vi "室内外单幅图像-视频预览.vi"() -> ()   [LabVIEW 2018]
doc: "This example shows how to open, read, and display an AVI file in NI Vision. The VI reads the frames per second property and plays the images back at the rate specified by the AVI file."
uses:
  <vilib>/Utility/error.llb/DialogType.ctl
panel:
  out "数值输入控件":i32
  in  "重新读取":bool
  out "视频的帧数：":u32
  out "Path":path
  out "添加的路径":path
  out "视频预览":T1(plugin-control)
  in  "Stop 2":bool
  out "Progress Bar 2":i32(slide) max=25 scale=-1.0..25.0
  in  "下一步":bool
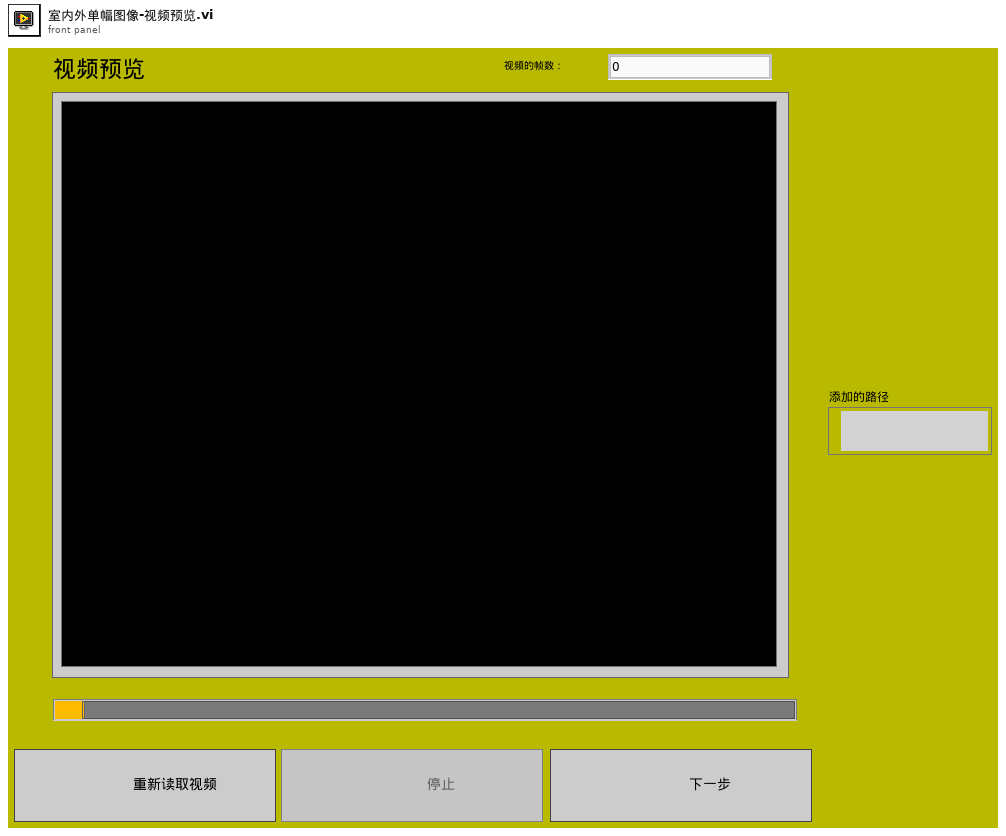
[diagram p1: front panel]
types:
  T1 = typedef "IMAQ Image.ctl" = refnum<image>
  T2 = enum8{"Enabled", "Disabled", "Disabled and Grayed Out"}
  T3 = enum32{"Invalid", "Standard", "Closed", "Hidden", "Minimized", "Maximized"}
  T4 = typedef "DialogType.ctl" = u16
  T5 = typedef "IMAQ AVI2 Refnum.ctl" = refnum<k20>
  T6 = typedef "Image Type" = u32
  T7 = cluster{"Width":u32, "Height":u32, "Frames Per Second":u32, "Codec":string, "Has Data":bool}
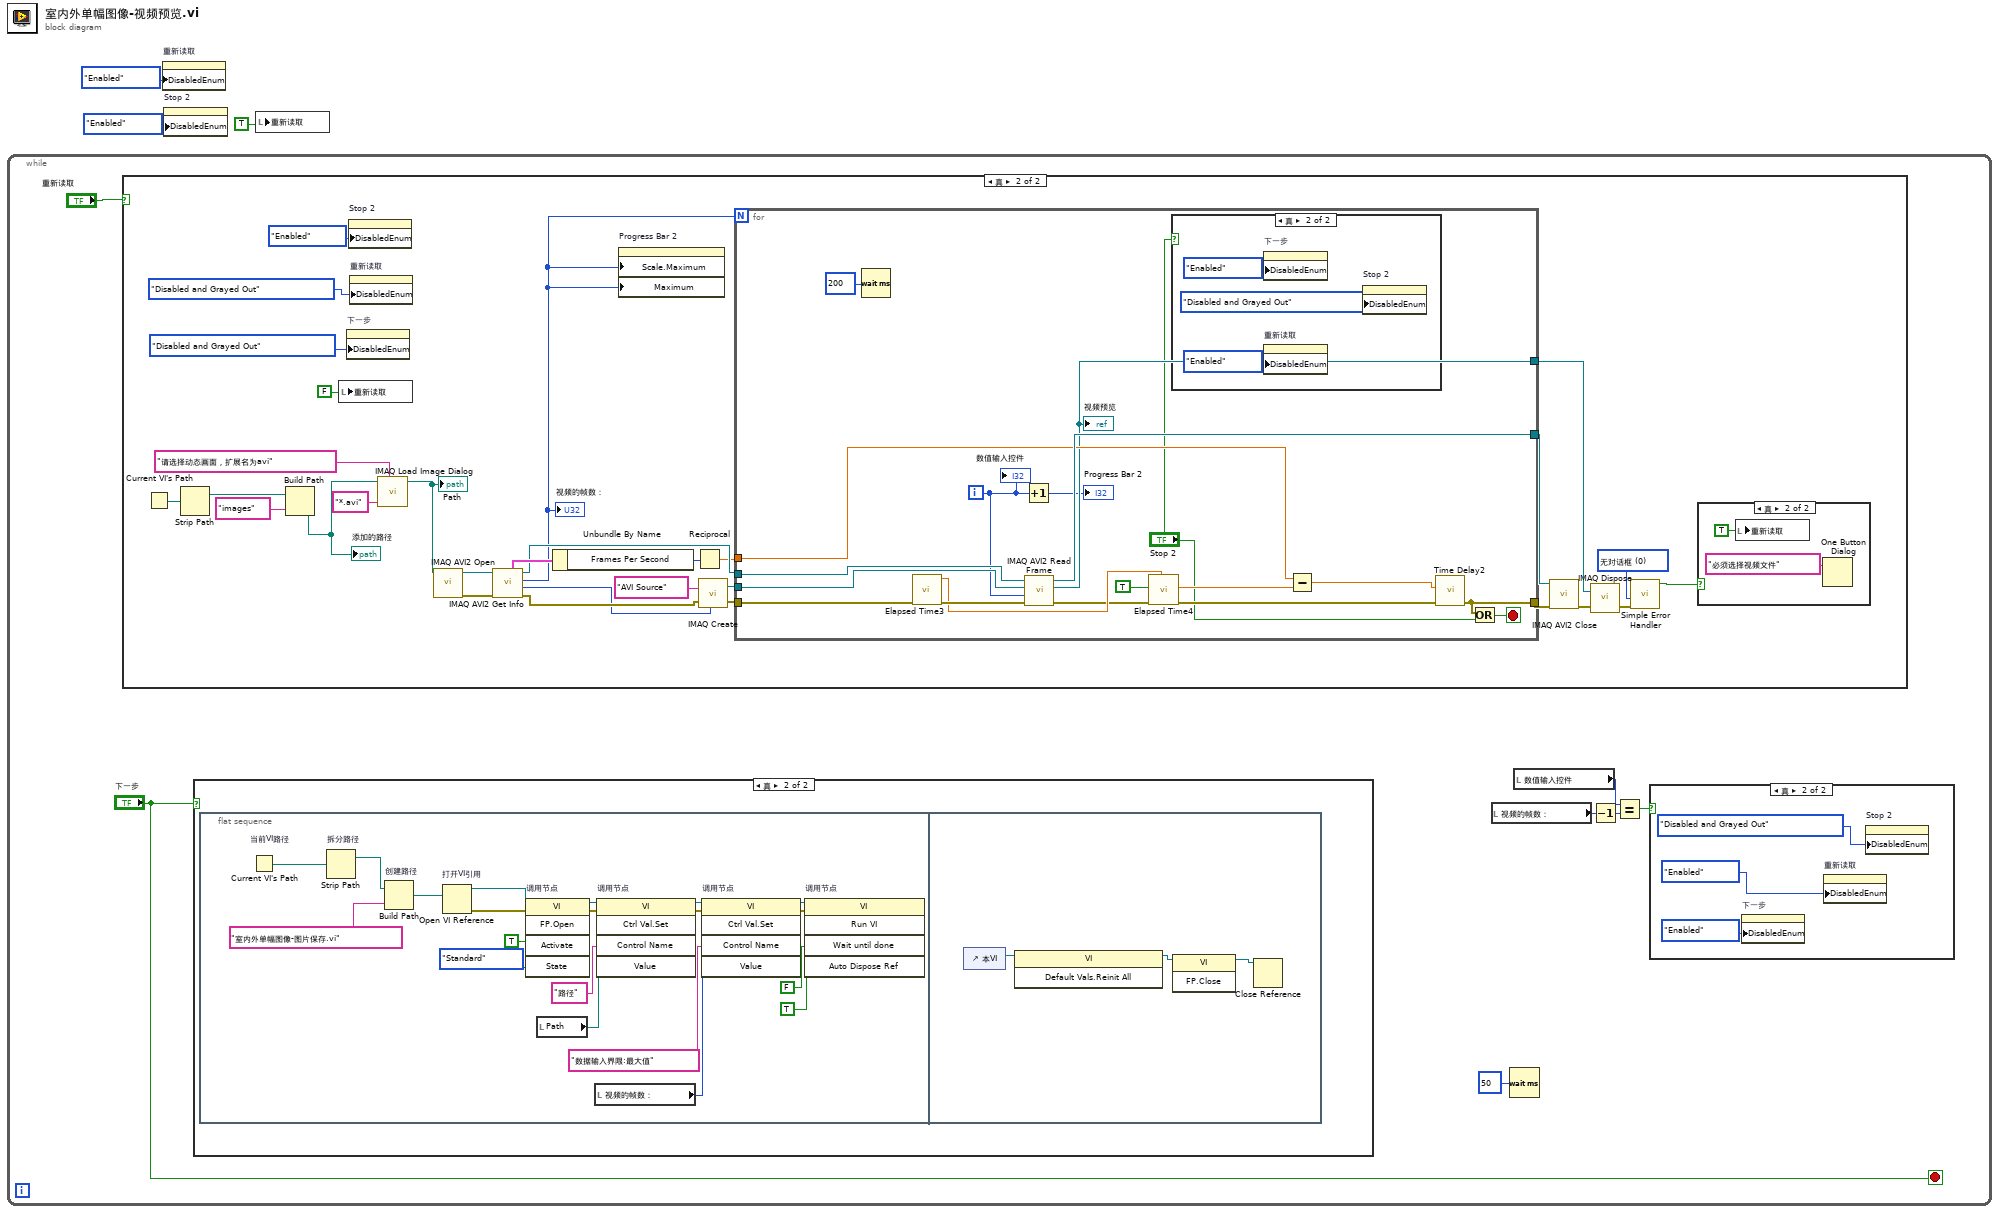
[diagram p0: block diagram]
diagram:
  n1 = while {
    stop <- "下一步" stop-if-true
    n2 = case shown="真" "重新读取" {
      frame False {
      }
      frame True {
        w19 = T4 0 items=["无对话框", "确定信息", "继续或停止信息", "确定信息＋警告", "继续/停止+警告"] ("type of dialog (OK msg:1)")
        n3 = Current VI's Path() -> (path=w23:path)
        n4 = Strip Path(path=w23) -> (stripped path=w22:path)  [unwired: 1 out]
        n5 = Build Path(base path=w22, name or relative path="images") -> (appended path=w26:path)
        "添加的路径" <- w26
        n6 = local write "重新读取"(FALSE ("布尔")) -> ()
        n7 = property on="下一步" class="Bool (严格)"("DisabledEnum"=T2."Disabled and Grayed Out" ("禁用")) -> ()  [unwired: 2 in, 2 out]
        n8 = property on="Stop 2" class="Bool"("DisabledEnum"=T2."Enabled" ("禁用")) -> ()  [unwired: 2 in, 2 out]
        n9 = property on="重新读取" class="Bool (严格)"("DisabledEnum"=T2."Disabled and Grayed Out" ("禁用")) -> ()  [unwired: 2 in, 2 out]
        n10 = call "IMAQ Load Image Dialog"("Prompt"="请选择动态画面，扩展名为avi" ("prompt"), "Pattern"="*.avi", "Start Path"=w26) -> ("Path"=w20:path)  [unwired: 6 in, 2 out]
        "Path" <- w20
        n11 = call "IMAQ AVI2 Open"("AVI File Path"=w20) -> ("error out"=w40:errorcluster, "AVI Refnum"=w39:T5)  [unwired: 2 in, 7 out]
        n12 = call "IMAQ AVI2 Get Info"("error in (no error)"=w40, "AVI Refnum"=w39) -> ("error out"=w36:errorcluster, "Image Type"=w30:T6, "Number of Frames"=w27:u32, "AVI Refnum (duplicate)"=w33:T5, "Frame Data"=w41:T7)  [unwired: 5 out]
        "视频的帧数：" <- w27
        n13 = Unbundle By Name(w41) -> ("Frames Per Second"=w29:u32)
        n14 = property on="Progress Bar 2" class="Slide (严格)"("Scale.Maximum"=w27, "Maximum"=w27) -> ()  [unwired: 2 in, 2 out]
        n15 = Reciprocal(x=w29) -> (1/x=w28:dbl)
        n16 = call "IMAQ Create"("Image Name"="AVI Source", "Image Type"=w30, "error in (no error)"=w36) -> ("New Image"=w34:T1, "error out"=w35:errorcluster)  [unwired: 1 in, 1 out]
        n17 = for {
          N: w27 -> [_]
          tunnel: w34 -> [w63]
          tunnel: [w62] -> w37
          tunnel: [w51] -> w38
          tunnel: w35 -> [w61]
          tunnel: w33 -> [w64]
          tunnel: [w57] -> w31
          tunnel: w28 -> [w59]
          i -> [w49]
          stop <- w50 stop-if-true
          n18 = Wait (ms)(milliseconds to wait=u32 200 ("等待时间（毫秒）")) -> ()  [unwired: 1 out]
          n19 = call "Elapsed Time3"("error in (no error)"=w61) -> ("Present (s)"=w56:dbl, "error out"=w60:errorcluster)  [unwired: 11 in, 6 out]
          n20 = Increment(x=w49) -> (x+1=→"Progress Bar 2":i32)
          n21 = call "IMAQ AVI2 Read Frame"("error in (no error)"=w60, "Frame Number"=w49, "Image"=w63, "AVI Refnum"=w64) -> ("error out"=w54:errorcluster, "Image Out"=w57:T1, "AVI Refnum (duplicate)"=w62:T5)  [unwired: 5 out]
          "视频预览" <- w57
          n22 = call "Elapsed Time4"("Reset"=TRUE, "error in (no error)"=w54, "Set Start Time (s)"=w56) -> ("Elapsed Time (s)"=w53:dbl, "error out"=w52:errorcluster)  [unwired: 9 in, 6 out]
          n23 = case shown="真" "Stop 2" {
            frame False {
            }
            frame True {
              n24 = property on="下一步" class="Bool (严格)"("DisabledEnum"=T2."Enabled" ("禁用")) -> ()  [unwired: 2 in, 2 out]
              n25 = property on="重新读取" class="Bool (严格)"("DisabledEnum"=T2."Enabled" ("禁用")) -> ()  [unwired: 2 in, 2 out]
              n26 = property on="Stop 2" class="Bool"("DisabledEnum"=T2."Disabled and Grayed Out" ("禁用")) -> ()  [unwired: 2 in, 2 out]
            }
          }
          n27 = Subtract(x=w59, y=w53) -> (x-y=w58:dbl)
          n28 = call "Time Delay2"("error in (no error)"=w52, "Delay Time (s)"=w58) -> ("error out"=w51:errorcluster)  [unwired: 9 in]
          n29 = Or(x=w51, y="Stop 2") -> (x .or. y?=w50:bool)
          "数值输入控件" <- w49
        }
        n30 = call "IMAQ AVI2 Close"("error in (no error)"=w38, "AVI Refnum"=w37) -> ("error out"=w32:errorcluster)  [unwired: 9 out]
        n31 = call "IMAQ Dispose"("Image"=w31, "error in (no error)"=w32) -> ("error out"=w42:errorcluster)  [unwired: 1 in, 3 out]
        n32 = call <vilib>:"Simple Error Handler.vi"("type of dialog (OK msg:1)"=w19, "error in (no error)"=w42) -> ("error?"=w14:bool)  [unwired: 7 out]
        n33 = case shown="真" w14 {
          frame False {
          }
          frame True {
            n34 = local write "重新读取"(TRUE ("布尔")) -> ()
            n35 = One Button Dialog(message="必须选择视频文件" ("消息")) -> ()  [unwired: 1 in, 1 out]
          }
        }
      }
    }
    n36 = case shown="真" "下一步" {
      frame False {
      }
      frame True {
        n37 = flat-sequence {
          frame #0 {
            n38 = Current VI's Path "当前VI路径"() -> (path=w83:path)
            n39 = Strip Path "拆分路径"(path=w83) -> (stripped path=w87:path)  [unwired: 1 out]
            n40 = Build Path "创建路径"(base path=w87, name or relative path="室内外单幅图像-图片保存.vi" ("名称或相对路径")) -> (appended path=w84:path)
            n41 = Open VI Reference "打开VI引用"(vi path=w84) -> (vi reference=w78:refnum<vi>, error out=w81:errorcluster)  [unwired: 5 in]
            n42 = invoke on="调用节点" class="VI" method="FP.Open"(reference=w78, error in=w81, "Activate"=TRUE ("激活？"), "State"=T3."Standard" ("状态")) -> (reference out=w73:refnum<vi>, error out=w69:errorcluster)  [unwired: 1 in, 3 out]
            n43 = local read "Path"() -> (w77:path)
            n44 = local read "视频的帧数："() -> (w75:u32)
            n45 = invoke on="调用节点" class="VI" method="Ctrl Val.Set"(reference=w73, error in=w69, "Control Name"="路径" ("控件名"), "Value"=w77) -> (reference out=w68:refnum<vi>, error out=w70:errorcluster)  [unwired: 1 in, 3 out]
            n46 = invoke on="调用节点" class="VI" method="Ctrl Val.Set"(reference=w68, error in=w70, "Control Name"="数据输入界限:最大值" ("控件名"), "Value"=w75) -> (reference out=w72:refnum<vi>, error out=w71:errorcluster)  [unwired: 1 in, 3 out]
            n47 = invoke on="调用节点" class="VI" method="Run VI"(reference=w72, error in=w71, "Wait until done"=FALSE ("结束前等待"), "Auto Dispose Ref"=TRUE ("自动销毁引用")) -> ()  [unwired: 1 in, 5 out]
          }
          frame #1 {
            n48 = control-ref of="本VI"() -> (w90:refnum<vi>)
            n49 = invoke class="VI" method="Default Vals.Reinit All"(reference=w90) -> (reference out=w89:refnum<vi>)  [unwired: 2 in, 2 out]
            n50 = invoke class="VI" method="FP.Close"(reference=w89) -> (reference out=w88:refnum<vi>)  [unwired: 2 in, 2 out]
            n51 = Close Reference(reference=w88) -> ()  [unwired: 1 in, 1 out]
          }
        }
      }
    }
    n52 = local read "视频的帧数："() -> (w6:u32)
    n53 = Wait (ms)(milliseconds to wait=u32 50 ("等待时间（毫秒）")) -> ()  [unwired: 1 out]
    n54 = local read "数值输入控件"() -> (w8:i32)
    n55 = Decrement(x=w6) -> (x-1=w5:u32)
    n56 = Equal?(x=w8, y=w5) -> (x = y?=w7:bool)
    n57 = case shown="真" w7 {
      frame False {
      }
      frame True {
        n58 = property on="下一步" class="Bool (严格)"("DisabledEnum"=T2."Enabled" ("禁用")) -> ()  [unwired: 2 in, 2 out]
        n59 = property on="重新读取" class="Bool (严格)"("DisabledEnum"=T2."Enabled" ("禁用")) -> ()  [unwired: 2 in, 2 out]
        n60 = property on="Stop 2" class="Bool"("DisabledEnum"=T2."Disabled and Grayed Out" ("禁用")) -> ()  [unwired: 2 in, 2 out]
      }
    }
  }
  n61 = property on="重新读取" class="Bool (严格)"("DisabledEnum"=T2."Enabled" ("禁用")) -> ()  [unwired: 2 in, 2 out]
  n62 = property on="Stop 2" class="Bool"("DisabledEnum"=T2."Enabled" ("禁用")) -> ()  [unwired: 2 in, 2 out]
  n63 = local write "重新读取"(TRUE ("布尔")) -> ()
